vi "DataBase_API_Init.vi"(8 "error in (no error)":errorcluster, 11 "DB Data":T1={"Cmd"=enum."WriteLog", "Temperature"=0.0, "Logs"=""}) -> (0 "error out":errorcluster)   [LabVIEW 2020]
uses:
  #typedef_DataBase.ctl
  Controller/#typedef_ControllerQueue_States.ctl
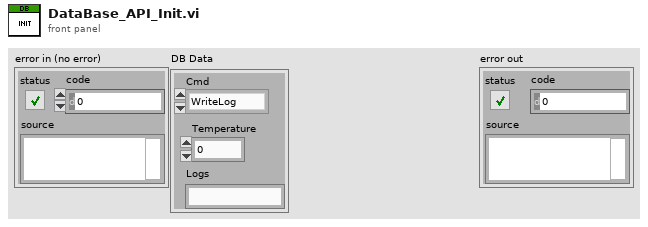
[diagram p1: front panel]
types:
  T1 = typedef "#typedef_DataBase.ctl" = cluster{"Cmd":enum16{"Idle", "WriteLog", "Exit"}, "Temperature":dbl, "Logs":string}
  T2 = typedef "#typedef_ControllerQueue_States.ctl" = enum16{"Obtain", "GetRef", "Enqueue", "EnqueueAtOpp", "GetStatus", "Flush", "Release"}
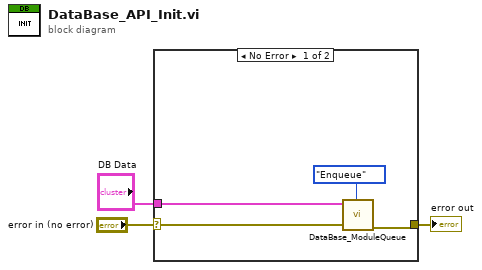
[diagram p0: block diagram]
diagram:
  n1 = case shown="No Error" "error in (no error)" {
    selector: "error in (no error)" -> [w5 w8]
    tunnel: [w7 w8] -> w2
    tunnel: "DB Data" -> [w4 _]
    frame No Error {
      n2 = call "DataBase_ModuleQueue.vi"(7:#typedef_ControllerQueue_States."Enqueue", "error in (no error)"=w5, "DB Data"=w4) -> ("error out"=w7:errorcluster)  [unwired: 6 in, 2 out]
    }
    frame Error {
    }
  }
  "error out" <- w2
